vi "Actions.vi"(8 "error in (no error)":errorcluster, 11 "MyAppController in":refnum<class "MyAppController.lvclass">) -> (0 "error out":errorcluster, 3 "MyAppController out":refnum<class "MyAppController.lvclass">)   [LabVIEW 2013, in "MyAppController.lvclass"]
uses:
  MyAppController.lvclass
  Framework/Controller/base/CONTROLLER.lvclass
  Framework/View/base/VIEW.lvclass
panel:
  out "Value":variant
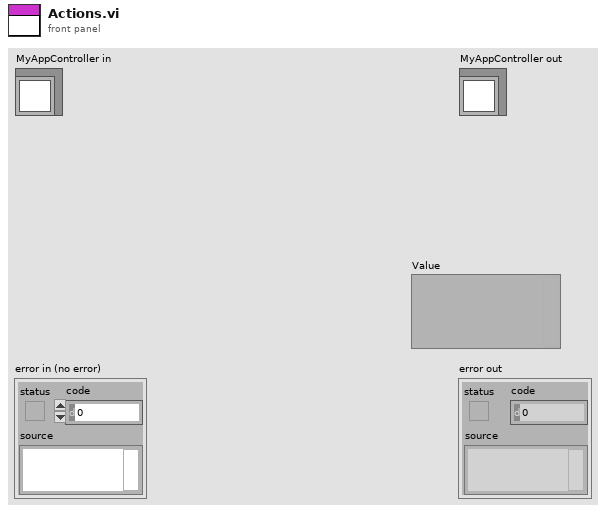
[diagram p1: front panel]
types:
  T1 = cluster{"CtlRef":refnum<vi>, "Name":string, "ClassName":string}
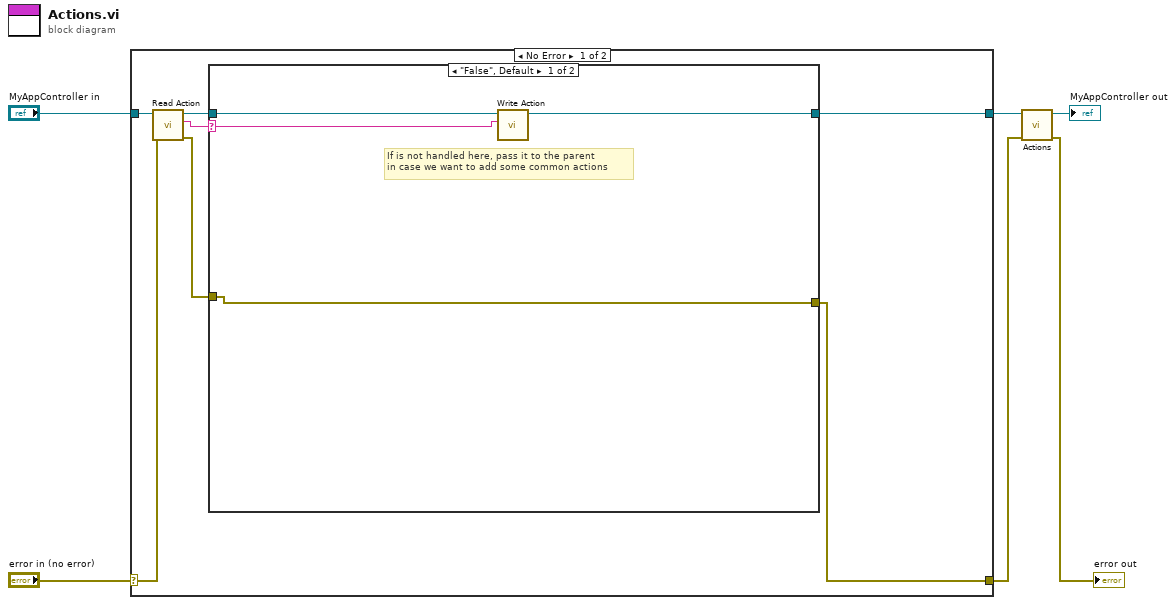
[diagram p0: block diagram]
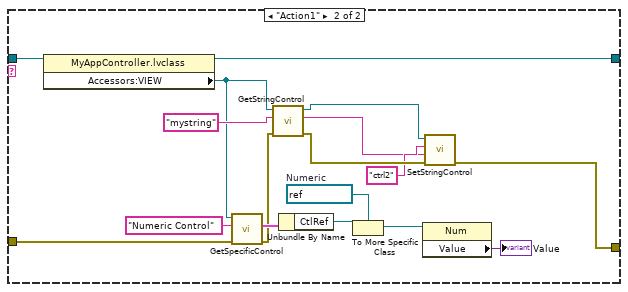
[diagram p2: hidden frame]
diagram:
  n1 = case shown="No Error" "error in (no error)" {
    selector: "error in (no error)" -> [w9 w36]
    tunnel: [w8 w36] -> w2
    tunnel: [w7 w35] -> w4
    tunnel: "MyAppController in" -> [w10 w35]
    frame No Error {
      n2 = call-dynamic "Read Action.vi"("error in (no error)"=w9, "CONTROLLER in"=w10) -> ("error out"=w13:errorcluster, "Action"=w11:string, "CONTROLLER out"=w12:refnum<class "MyAppController.lvclass">)  [unwired: 7 in]
      n3 = case shown="\"False\", Default" w11 {
        selector: w11 -> [w14 _]
        tunnel: w12 -> [w17 w22]
        tunnel: [w15 w21] -> w7
        tunnel: w13 -> [w16 w20]
        tunnel: [w16 w18] -> w8
        frame "False", Default {
          # "If is not handled here, pass it to the parent\nin case we want to add some common actions"
          n4 = call-dynamic "Write Action.vi"("Action"=w14, "CONTROLLER in"=w17) -> ("CONTROLLER out"=w15:refnum<class "MyAppController.lvclass">)  [unwired: 8 in, 1 out]
        }
        frame "Action1" {
          w25 = refnum<vi> refnum  # Numeric
          n5 = property class="MyAppController.lvclass"(reference=w22) -> (reference out=w21:refnum<class "MyAppController.lvclass">, "Accessors:VIEW"=w29:refnum<class "VIEW.lvclass">)  [unwired: 1 in, 1 out]
          n6 = call "GetSpecificControl.vi"("error in (no error)"=w20, "Name"="Numeric Control", "VIEW in"=w29) -> ("error out"=w19:errorcluster, "output cluster"=w27:T1)  [unwired: 6 in, 1 out]
          n7 = call "GetStringControl.vi"("error in (no error)"=w19, "Name"="mystring", "VIEW in"=w29) -> ("error out"=w34:errorcluster, "Text.Text"=w30:string, "VIEW out"=w32:refnum<class "VIEW.lvclass">)  [unwired: 6 in]
          n8 = Unbundle By Name(w27) -> ("CtlRef"=w26:refnum<vi>)
          n9 = To More Specific Class(target class=w25, reference=w26) -> (specific class reference=w24:refnum<vi>)  [unwired: 1 in, 1 out]
          n10 = property class="Num"(reference=w24) -> ("Value"=→"Value":variant)  [unwired: 1 in, 2 out]
          n11 = call "SetStringControl.vi"("error in (no error)"=w34, "Text.Text"=w30, "Name"="ctrl2", "VIEW in"=w32) -> ("error out"=w18:errorcluster)  [unwired: 6 in, 1 out]
        }
      }
    }
    frame Error {
    }
  }
  n12 = call-parent "Actions.vi"("error in (no error)"=w2, "CONTROLLER in"=w4) -> ("error out"=→"error out":errorcluster, "CONTROLLER out"=→"MyAppController out":refnum<class "MyAppController.lvclass">)  [unwired: 8 in]
